vi "ColorWheelSpinSense.vi"(1 "Color":T1, 2 "Reset":bool) -> (0 "x+y":dbl)   [LabVIEW 2019]
uses:
  TypeDefs/ControlPanelColor.ctl
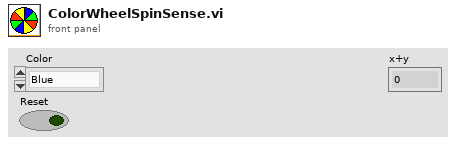
[diagram p1: front panel]
types:
  T1 = typedef "ControlPanelColor.ctl" = enum16{"Blue", "Green", "Red", "Yellow", "Unknown"}
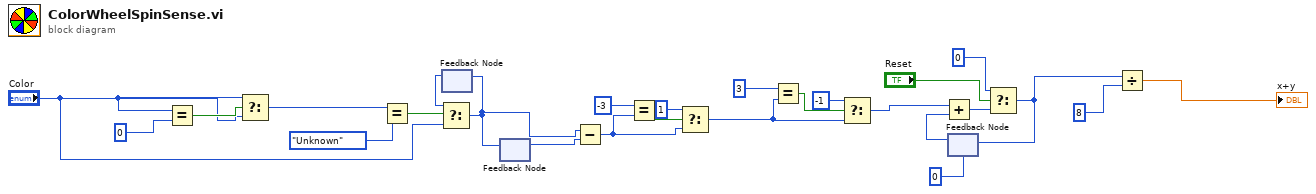
[diagram p0: block diagram]
diagram:
  n1 = Equal?(x="Color", y=0) -> (x = y?=w7:bool)
  n2 = Select(t="Color", s=w7, f="Color") -> (s? t:f=w9:T1)
  n3 = Equal?(x=w9, y=ControlPanelColor."Unknown") -> (x = y?=w25:bool)
  n4 = feedback #1() -> (w24:T1)  [unwired: 1 in]
  n5 = Select(t=w24, s=w25, f="Color") -> (s? t:f=w23:T1)
  n6 = feedback-in #1(w23) -> ()
  n7 = feedback-in #2(w23) -> ()
  n8 = feedback #2() -> (w22:T1)  [unwired: 1 in]
  n9 = Subtract(x=w23, y=w22) -> (x-y=w18:i8)
  n10 = Equal?(x=i8 -3, y=w18) -> (x = y?=w19:bool)
  n11 = Select(t=i8 1, s=w19, f=w18) -> (s? t:f=w14:i8)
  n12 = Equal?(x=i8 3, y=w14) -> (x = y?=w16:bool)
  n13 = Select(t=i8 -1, s=w16, f=w14) -> (s? t:f=w13:i8)
  n14 = feedback #3(i8 0) -> (w5:i8)
  n15 = Add(x=w13, y=w5) -> (x+y=w4:i8)
  n16 = Select(t=i8 0, s="Reset", f=w4) -> (s? t:f=w1:i8)
  n17 = feedback-in #3(w1) -> ()
  n18 = Divide(x=w1, y=i8 8) -> (x/y=→"x+y":dbl)
